vi "PH_AxisGUI_BaseClass.set Settings to GUI.vi"(4 "error in (no error)":errorcluster, 5 "No link?":bool, 6 "Axis Settings":T1, 7 "GUI Ref Settings":refnum<vi>) -> (0 "error out":errorcluster)   [LabVIEW 2014, in "PH_AxisGUI_BaseClass.lvlib"]
doc: "This VI sets the current axis settings to the GUI."
uses:
  PH_AxisGUI_BaseClass.lvlib
  PH_Stepmotor_BaseClass/PH_Stepmotor_BaseClass.Axis Settings.ctl
  PH_Stepmotor_BaseClass/PH_Stepmotor_BaseClass.Motor Type.ctl
  PH_Stepmotor_BaseClass/PH_Stepmotor_BaseClass.lvlib
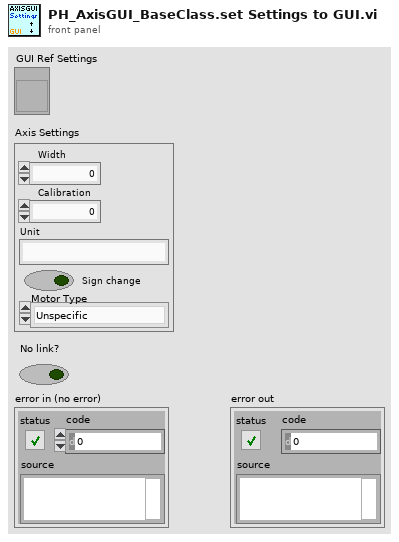
[diagram p1: front panel]
types:
  T1 = typedef "PH_Stepmotor_BaseClass.lvlib/PH_Stepmotor_BaseClass.Axis Settings.ctl" = cluster{"Sign change":bool, "Width":dbl, "Calibration":dbl, "Unit":string, "Motor Type":T2, "Unit Width":string, "Unit CF":string}
  T2 = typedef "PH_Stepmotor_BaseClass.lvlib/PH_Stepmotor_BaseClass.Motor Type.ctl" = enum16{"Unspecific", "OWIS 49.120.2633", "OWIS 49.060.1033", "OWIS 43.040.2558", "Diamond Motion 2200 series", "OWIS 49.120.266B.MV6", "Calorimeter", "Linear Stage 1", "MICOS VT-80", "MICOS VT-80 S", "Standa Rotstage nt0.95A", "PUF RA 320.200", "PUF RA 800.200", "PUF RA 800.400", "PUF RA 400.50", "1324.nn.800.50", "1324.n9c.800.50", "1324.nn.320.200", "1324.nn.400.200", "1324.nn.800.200", "1324.nn.400.50", "1324.8c9c.800.50", "1324.8c9c.400.200"}
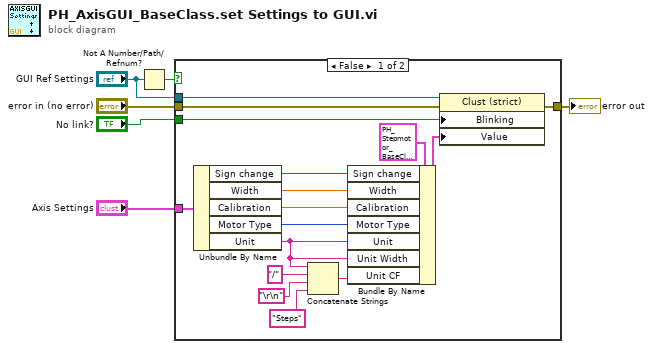
[diagram p0: block diagram]
diagram:
  n1 = Not A Number/Path/Refnum?(number/path/refnum="GUI Ref Settings") -> (NaN/Path/Refnum?=w3:bool)
  n2 = case shown="False" w3 {
    tunnel: "GUI Ref Settings" -> [w21 _]
    tunnel: "error in (no error)" -> [w20 w23]
    tunnel: "Axis Settings" -> [w19 _]
    tunnel: [w17 w23] -> w5
    tunnel: "No link?" -> [w18 _]
    frame False {
      n3 = Unbundle By Name(w19) -> ("Sign change"=w14:bool, "Width"=w13:dbl, "Calibration"=w12:dbl, "Motor Type"=w11:T2, "Unit"=w10:string)
      n4 = Concatenate Strings(w10, "/", "\r\n", "Steps") -> (w9:string)
      n5 = Bundle By Name(cluster=T1 {"Sign change"=FALSE, "Width"=0.0, "Calibration"=0.0, "Unit"="Steps", "Motor Type"=enum."Unspecific", "Unit Width"="Steps", "Unit CF"="Steps/Steps"} ("Value"), "Sign change"=w14, "Width"=w13, "Calibration"=w12, "Motor Type"=w11, "Unit"=w10, "Unit Width"=w10, "Unit CF"=w9) -> (w15:T1)
      n6 = property class="Clust (strict)"(reference=w21, error in=w20, "Blinking"=w18, "Value"=w15) -> (error out=w17:errorcluster)  [unwired: 1 out]
    }
    frame True {
    }
  }
  "error out" <- w5
